vi "PWM Pulsate.vi"() -> ()   [LabVIEW 2020, in "CTI-Scratchpad.lvlib"]
uses:
  CTI-Scratchpad.lvlib
  CTI/GPIO Number.ctl
  CTI/Session/Session.lvclass
  <vilib>/ptbypt/NI_PtbyPt.lvlib
  CTI/VisaComms/VisaComms.lvclass
  CTI/PWM/PWM.lvclass
  CTI/CTI.lvlib
panel:
  in  "Speed":i32(slide) scale=1000.0..1.0
  in  "stop":bool
  out "Act. Duty":sgl format="%_6f"
  in  "Port":refnum<visa-resource-name>="COM3"
  in  "Channel":T1
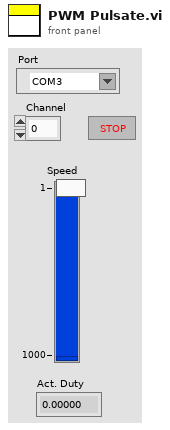
[diagram p1: front panel]
types:
  T1 = typedef "CTI.lvlib/GPIO Number.ctl" = i8
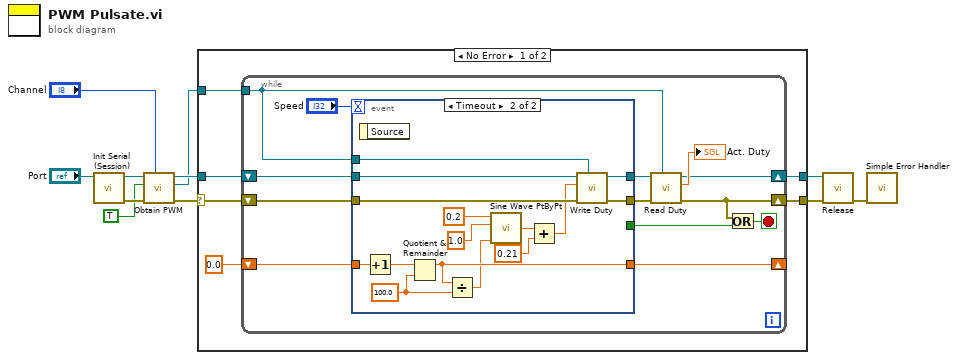
[diagram p0: block diagram]
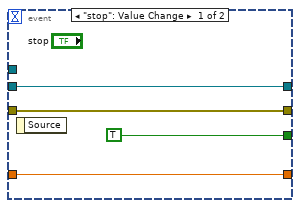
[diagram p2: hidden frame]
diagram:
  n1 = call "Init Serial (Session).vi"("VISA resource name in"="Port") -> ("error out"=w9:errorcluster, "Session"=w10:refnum<class "Session.lvclass">)  [unwired: 9 in]
  n2 = call "Obtain PWM.vi"("GPIO #"="Channel", "error in (no error)"=w9, "Enable (F)"=TRUE, "Session in"=w10) -> ("error out"=w8:errorcluster, "PWM"=w1:refnum<class "PWM.lvclass">, "Session out"=w7:refnum<class "Session.lvclass">)  [unwired: 5 in]
  n3 = case shown="No Error" w8 {
    selector: w8 -> [w16 w50]
    tunnel: w7 -> [w17 w51]
    tunnel: [w15 w51] -> w5
    tunnel: [w14 w50] -> w6
    tunnel: w1 -> [w13 _]
    frame No Error {
      n4 = while {
        shift-right: [w22] -> w15
        shift-left: w17 -> [w29]
        shift-right: [w21] -> w14
        shift-left: w16 -> [w28]
        tunnel: w13 -> [w18]
        shift-right: [w19] -> _
        shift-left: 0.0 -> [w20]
        stop <- w30 stop-if-true
        n5 = event shown="[1] Timeout" {
          selector: _ -> [_ _]
          dyn-events: _ -> [_ _]
          timeout: "Speed" -> [_ _]
          tunnel: [w34 w42] -> w26
          tunnel: w29 -> [w34 w47]
          tunnel: [w33 w43] -> w25
          tunnel: w28 -> [w33 w46]
          tunnel: [TRUE _] -> w27
          tunnel: w20 -> [w31 w41]
          tunnel: [w31 w38] -> w19
          tunnel: w18 -> [_ w36]
          event "stop": Value Change {
            n6 = event-data() -> ()  [unwired: 1 in, 1 out]
          }
          event Timeout {
            w39 = 100.0 ("frequency")
            n7 = event-data() -> ()  [unwired: 1 in, 1 out]
            n8 = Increment(x=w41) -> (x+1=w40:dbl)
            n9 = Quotient & Remainder(x=w40, y=w39) -> (x-y*floor(x/y)=w38:dbl)  [unwired: 1 out]
            n10 = Divide(x=w38, y=w39) -> (x/y=w37:dbl)
            n11 = call <vilib>:"Sine Wave PtByPt.vi"("time"=w37, "frequency"=1.0, "amplitude"=0.2) -> ("sine wave"=w45:dbl)  [unwired: 1 in]
            n12 = Add(x=w45, y=0.21) -> (x+y=w35:dbl)
            n13 = call "Write Duty.vi"("PWM"=w36, "error in (no error)"=w46, "Duty % (0-1)"=w35, "Session In"=w47) -> ("error out"=w43:errorcluster, "Session Out"=w42:refnum<class "Session.lvclass">)  [unwired: 6 in]
          }
        }
        n14 = call "Read Duty.vi"("PWM"=w18, "error in (no error)"=w25, "Session In"=w26) -> ("error out"=w21:errorcluster, "Duty % (0-1)"=→"Act. Duty":sgl, "Session Out"=w22:refnum<class "Session.lvclass">)  [unwired: 6 in]
        n15 = Or(x=w21, y=w27) -> (x .or. y?=w30:bool)
      }
    }
    frame Error {
    }
  }
  n16 = call-dynamic "Release.vi"("error in (no error)"=w6, "Session in"=w5) -> ("error out"=w4:errorcluster)  [unwired: 9 in]
  n17 = call <vilib>:"Simple Error Handler.vi"("error in (no error)"=w4) -> ()  [unwired: 4 in, 5 out]
